vi "Scene Light Event.vi"(4 "Light Action":enum16{"Update", "Remove", "Nothing"}(ring), 8 "error in (no error)":errorcluster, 9 "Object Cluster In":T1, 11 "3D Plot.lvclass in":refnum<class "3D Plot.lvclass">) -> (0 "error out":errorcluster, 1 "Object Cluster Out":T1, 3 "3D Plot.lvclass out":refnum<class "3D Plot.lvclass">)   [LabVIEW 2020, in "3D Plot.lvclass"]
uses:
  3D Plot.lvclass
  Object Cluster.ctl
  3D Plot.lvclass/3D Plot.ctl
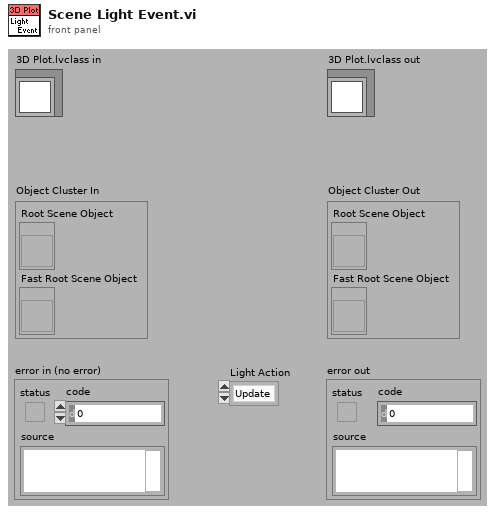
[diagram p1: front panel]
types:
  T1 = typedef "3D Plot.lvclass/Object Cluster.ctl" = cluster{"Root Scene Object":refnum<vi>, "Fast Root Scene Object":refnum<vi>}
  T2 = typedef "3D Plot.lvclass/Light Property.ctl" = cluster{"Enable Lighting?":bool, "Ambient Color":u32, "Light Array":T3[]}
  T3 = typedef "3D Plot.lvclass/Light Specific.ctl" = cluster{"Enable Light?":bool, "Light Color":u32, "Light Latitude":sgl, "Light Longitude":sgl, "Light Distance":sgl, "Attenuation":enum16{"None", "Linear", "Quadratic"}}
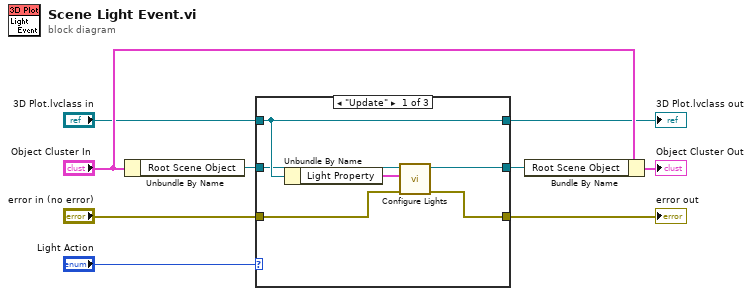
[diagram p0: block diagram]
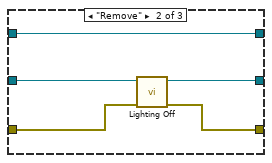
[diagram p2: hidden frame]
diagram:
  n1 = Unbundle By Name("Object Cluster In") -> ("Root Scene Object"=w8:refnum<vi>)
  n2 = case shown="\"Update\"" "Light Action" {
    tunnel: "error in (no error)" -> [w10 w17 w22]
    tunnel: w8 -> [w11 w19 w21]
    tunnel: "3D Plot.lvclass in" -> [w12 w20 w23]
    tunnel: [w12 w20 w23] -> w4
    tunnel: [w14 w18 w21] -> w3
    tunnel: [w13 w16 w22] -> w2
    frame "Update" {
      n3 = Unbundle By Name(w12) -> ("Light Property"=w15:T2)
      n4 = call "Configure Lights.vi"("error in (no error)"=w10, "Light Property"=w15, "Root Object In"=w11) -> ("error out"=w13:errorcluster, "Root Object Out"=w14:refnum<vi>)  [unwired: 7 out]
    }
    frame "Remove" {
      n5 = call "Lighting Off.vi"("error in (no error)"=w17, "Root Object In"=w19) -> ("error out"=w16:errorcluster, "Root Object Out"=w18:refnum<vi>)  [unwired: 8 out]
    }
    frame "Nothing", Default {
    }
  }
  "error out" <- w2
  "3D Plot.lvclass out" <- w4
  n6 = Bundle By Name(cluster="Object Cluster In", "Root Scene Object"=w3) -> (→"Object Cluster Out":T1)
